vi "Force Array To Size.vi"(5 "Default Value":dbl format="%.2f", 6 "Boolean Array In":bool[](array[boolean]), 7 "# Elements":i32, 8 "String Array In":string[](array[string]), 9 "2D U8 Array In":u8[][](array[numeric]), 10 "DBL Array In":dbl[](array[numeric]) format="%.2f", 11 "I32 Array In":i32[](array[numeric])) -> (0 "String Array Out":string[](array[string]), 1 "2D U8 Array Out":u8[][](array[numeric]), 2 "DBL Array Out":dbl[](array[numeric]) format="%.2f", 3 "I32 Array Out":i32[](array[numeric]), 4 "Boolean Array Out":bool[](array[boolean]))   [LabVIEW 2024]
panel:
  # "If input array has the specified number of elements, it is not changed.\nIf input array has more than the specified number of elements, the extra elements are removed from the end.\nIf input array has less than specified number of elements, it is padded using the default value."
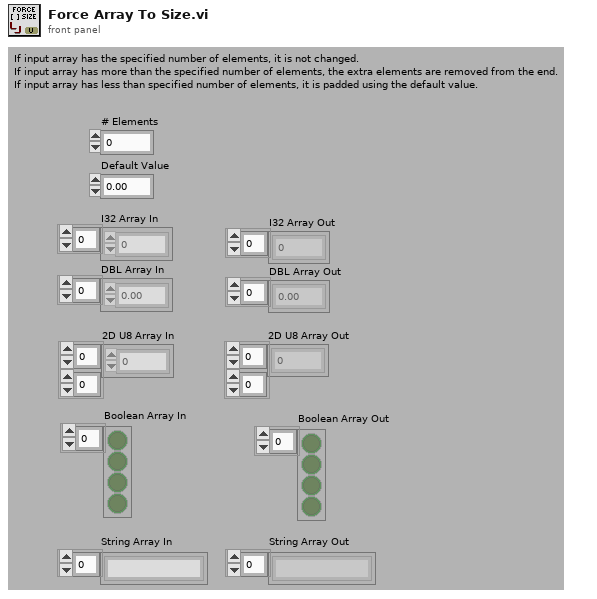
[diagram p1: front panel]
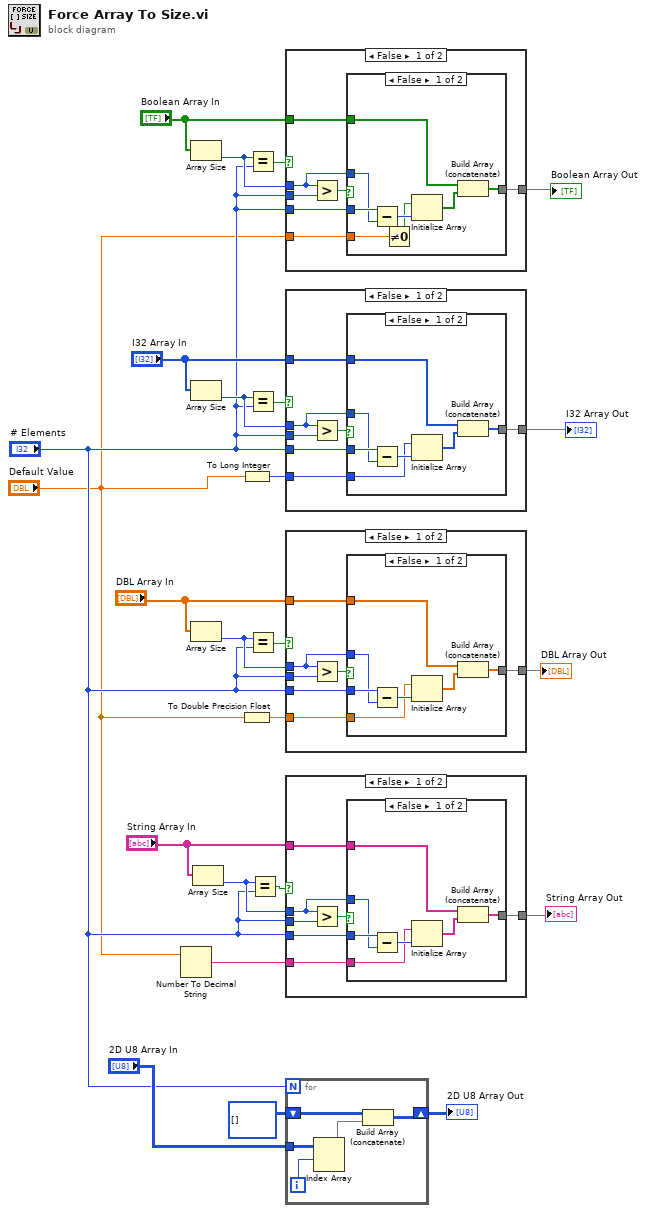
[diagram p0: block diagram]
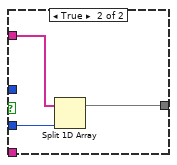
[diagram p2: hidden frame]
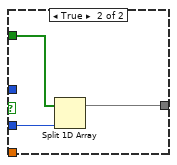
[diagram p4: hidden frame]
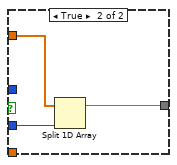
[diagram p6: hidden frame]
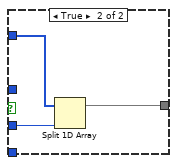
[diagram p8: hidden frame]
diagram:
  n1 = Number To Decimal String(number="Default Value") -> (decimal integer string=w2:string)  [unwired: 1 in]
  n2 = Array Size(array="Boolean Array In") -> (size(s)=w10:i32)
  n3 = Array Size(array="I32 Array In") -> (size(s)=w24:i32)
  n4 = Array Size(array="DBL Array In") -> (size(s)=w17:i32)
  n5 = Array Size(array="String Array In") -> (size(s)=w5:i32)
  n6 = To Long Integer(number="Default Value") -> (32bit integer=w21:i32)
  n7 = To Double Precision Float(number="Default Value") -> (double precision float=w19:dbl)
  n8 = Equal?(x=w10, y="# Elements") -> (x = y?=w11:bool)
  n9 = Equal?(x=w24, y="# Elements") -> (x = y?=w23:bool)
  n10 = Equal?(x=w17, y="# Elements") -> (x = y?=w18:bool)
  n11 = Equal?(x=w5, y="# Elements") -> (x = y?=w7:bool)
  n12 = case shown="False" w11 {
    tunnel: w10 -> [w26 _]
    tunnel: "# Elements" -> [w31 _]
    tunnel: "# Elements" -> [w29 _]
    tunnel: "Boolean Array In" -> [w28 w43]
    tunnel: [w27 w43] -> w8
    tunnel: "Default Value" -> [w25 _]
    frame False {
      n13 = Greater?(x=w26, y=w31) -> (0:w30:bool)
      n14 = case shown="False" w30 {
        tunnel: w29 -> [w39 w42]
        tunnel: w28 -> [w35 w41]
        tunnel: [w34 w40] -> w27
        tunnel: w26 -> [w38 _]
        tunnel: w25 -> [w33 _]
        frame False {
          n15 = Subtract(x=w39, y=w38) -> (x-y=w37:i32)
          n16 = Not Equal To 0?(x=w33) -> (x != 0?=w32:bool)
          n17 = Initialize Array(w32, w37) -> (w36:bool[])
          n18 = Build Array (concatenate)(w35, w36) -> (w34:bool[])
        }
        frame True {
          n19 = Split 1D Array(array=w41, index=w42) -> (first subarray=w40:bool[])  [unwired: 1 out]
        }
      }
    }
    frame True {
    }
  }
  "Boolean Array Out" <- w8
  n20 = case shown="False" w23 {
    tunnel: w24 -> [w45 _]
    tunnel: "# Elements" -> [w50 _]
    tunnel: "# Elements" -> [w48 _]
    tunnel: "I32 Array In" -> [w47 w61]
    tunnel: [w46 w61] -> w20
    tunnel: w21 -> [w44 _]
    frame False {
      n21 = Greater?(x=w45, y=w50) -> (0:w49:bool)
      n22 = case shown="False" w49 {
        tunnel: w48 -> [w57 w60]
        tunnel: w47 -> [w52 w59]
        tunnel: [w51 w58] -> w46
        tunnel: w45 -> [w56 _]
        tunnel: w44 -> [w54 _]
        frame False {
          n23 = Subtract(x=w57, y=w56) -> (x-y=w55:i32)
          n24 = Initialize Array(w54, w55) -> (w53:i32[])
          n25 = Build Array (concatenate)(w52, w53) -> (w51:i32[])
        }
        frame True {
          n26 = Split 1D Array(array=w59, index=w60) -> (first subarray=w58:i32[])  [unwired: 1 out]
        }
      }
    }
    frame True {
    }
  }
  "I32 Array Out" <- w20
  n27 = case shown="False" w18 {
    tunnel: w17 -> [w63 _]
    tunnel: "# Elements" -> [w68 _]
    tunnel: "# Elements" -> [w66 _]
    tunnel: "DBL Array In" -> [w65 w79]
    tunnel: [w64 w79] -> w16
    tunnel: w19 -> [w62 _]
    frame False {
      n28 = Greater?(x=w63, y=w68) -> (0:w67:bool)
      n29 = case shown="False" w67 {
        tunnel: w66 -> [w75 w78]
        tunnel: w65 -> [w70 w77]
        tunnel: [w69 w76] -> w64
        tunnel: w63 -> [w74 _]
        tunnel: w62 -> [w72 _]
        frame False {
          n30 = Subtract(x=w75, y=w74) -> (x-y=w73:i32)
          n31 = Initialize Array(w72, w73) -> (w71:dbl[])
          n32 = Build Array (concatenate)(w70, w71) -> (w69:dbl[])
        }
        frame True {
          n33 = Split 1D Array(array=w77, index=w78) -> (first subarray=w76:dbl[])  [unwired: 1 out]
        }
      }
    }
    frame True {
    }
  }
  "DBL Array Out" <- w16
  n34 = case shown="False" w7 {
    tunnel: w5 -> [w81 _]
    tunnel: "# Elements" -> [w86 _]
    tunnel: "# Elements" -> [w84 _]
    tunnel: "String Array In" -> [w83 w97]
    tunnel: [w82 w97] -> w1
    tunnel: w2 -> [w80 _]
    frame False {
      n35 = Greater?(x=w81, y=w86) -> (0:w85:bool)
      n36 = case shown="False" w85 {
        tunnel: w84 -> [w93 w96]
        tunnel: w83 -> [w88 w95]
        tunnel: [w87 w94] -> w82
        tunnel: w81 -> [w92 _]
        tunnel: w80 -> [w90 _]
        frame False {
          n37 = Subtract(x=w93, y=w92) -> (x-y=w91:i32)
          n38 = Initialize Array(w90, w91) -> (w89:string[])
          n39 = Build Array (concatenate)(w88, w89) -> (w87:string[])
        }
        frame True {
          n40 = Split 1D Array(array=w95, index=w96) -> (first subarray=w94:string[])  [unwired: 1 out]
        }
      }
    }
    frame True {
    }
  }
  "String Array Out" <- w1
  n41 = for {
    N: "# Elements" -> [_]
    shift-right: [w98] -> w13
    shift-left: u8[][] [] -> [w99]
    tunnel: "2D U8 Array In" -> [w102]
    i -> [w101]
    n42 = Index Array(array=w102, index (row)=w101) -> (element=w100:u8[])  [unwired: 1 in]
    n43 = Build Array (concatenate)(w99, w100) -> (w98:u8[][])
  }
  "2D U8 Array Out" <- w13
